vi "tokenize.vi"(11 "input string":string="(+ hello (/ 2 3 4))") -> (3 "Tokens":string[](array[string]))   [LabVIEW 2020]
uses:
  <vilib>/regexp/Match Regular Expression.xnode
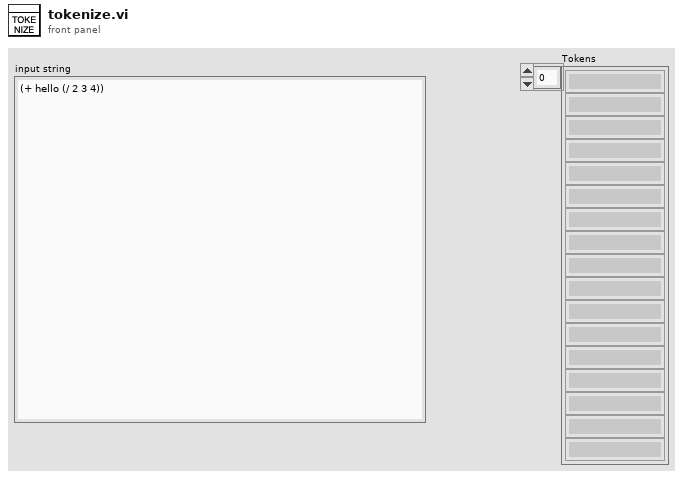
[diagram p1: front panel]
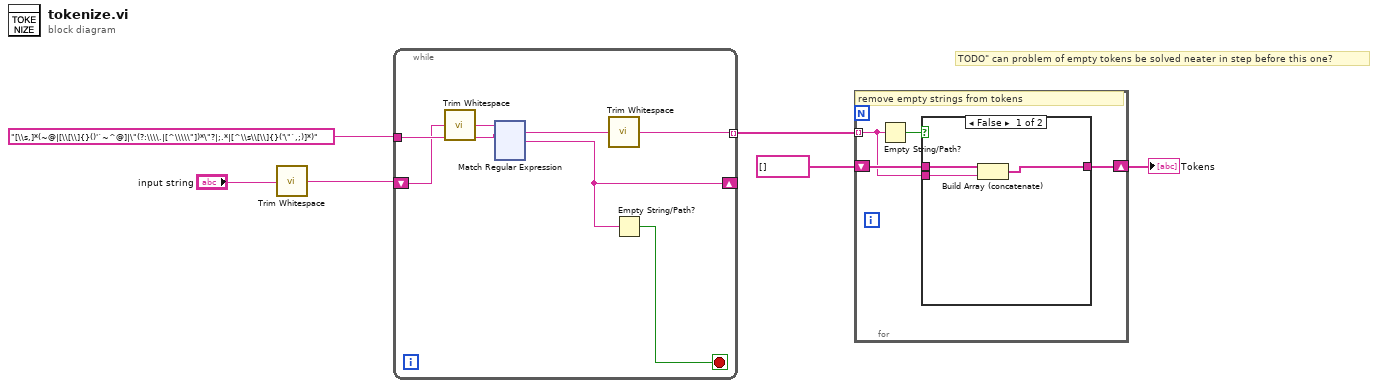
[diagram p0: block diagram]
diagram:
  # "TODO\" can problem of empty tokens be solved neater in step before this one?"
  n1 = call <vilib>:"Trim Whitespace.vi"("string"="input string") -> ("trimmed string"=w4:string)  [unwired: 1 in]
  n2 = while {
    tunnel: "[\\s,]*(~@|[\\[\\]{}()'`~^@]|\"(?:\\\\.|[^\\\\\"])*\"?|;.*|[^\\s\\[\\]{}('\"`,;)]*)" ("regular expression") -> [w9]
    tunnel: [w10] -> w3 mode=indexing
    shift-right: [w13] -> _
    shift-left: w4 -> [w8]
    stop <- w12 stop-if-true
    n3 = call <vilib>:"Trim Whitespace.vi"("string"=w8) -> ("trimmed string"=w7:string)  [unwired: 1 in]
    n4 = xnode "Match Regular Expression"("input string"=w7, "regular expression"=w9) -> ("whole match"=w11:string, "after match"=w13:string)  [unwired: 4 in, 3 out]
    n5 = call <vilib>:"Trim Whitespace.vi"("string"=w11) -> ("trimmed string"=w10:string)  [unwired: 1 in]
    n6 = Empty String/Path?(string/path=w13) -> (empty?=w12:bool)
  }
  n7 = for {
    tunnel: w3 -> [w131] mode=indexing
    shift-right: [w132] -> w1
    shift-left: string[] [] -> [w133]
    # "remove empty strings from tokens"
    n8 = Empty String/Path?(string/path=w131) -> (empty?=w134:bool)
    n9 = case shown="False" w134 {
      tunnel: [w136 w138] -> w132
      tunnel: w133 -> [w137 w138]
      tunnel: w131 -> [w135 _]
      frame False {
        n10 = Build Array (concatenate)(w137, w135) -> (w136:string[])
      }
      frame True {
      }
    }
  }
  "Tokens" <- w1
